vi "Ventil Setzen.vi"(8 "Error In":errorcluster caption="Fehler (Eingang)", 10 "Thermostat in %":dbl, 11 "Verbindungs-ID in":refnum<k16>) -> (0 "Error Out":errorcluster caption="Fehler (Ausgang)", 3 "Verbindungs-ID out":refnum<k16>)   [LabVIEW 2024, in "Thermostat Treiber.lvlib"]
doc: "Dieses VI sendet einen neuen Sollwert zu dem Thermotat. Der Therostat erlaubt nur Werte zweischen 0 und 100%. Wenn der Wert außerhalb des Bereiches liegt, liefert die Funktion einen fehler als Rückgabe."
uses:
  Thermostat Treiber.lvlib
  SubVIs/Simulation Share.vi
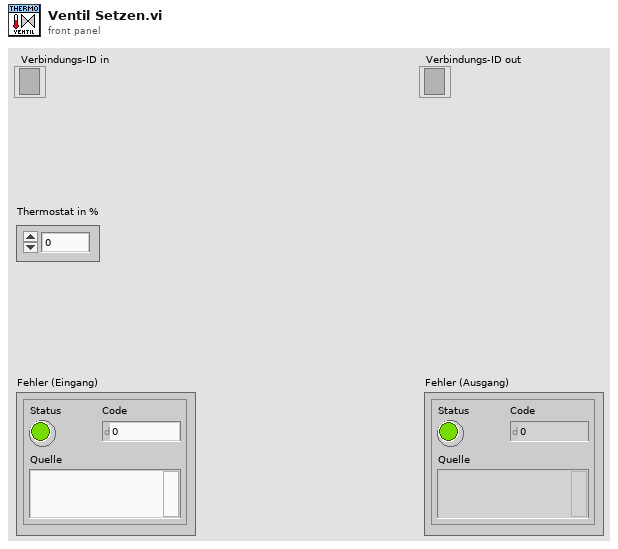
[diagram p1: front panel]
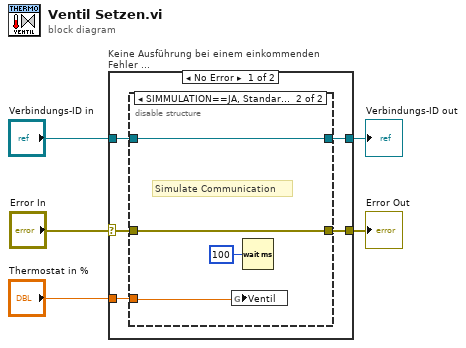
[diagram p0: block diagram]
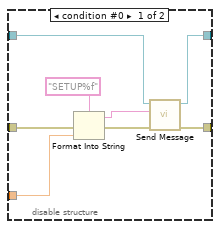
[diagram p2: hidden frame]
diagram:
  n1 = case "Keine Ausführung bei einem einkommenden Fehler ..." shown="No Error" "Error In" {
    selector: "Error In" -> [w10 w24]
    tunnel: [w7 w24] -> w4
    tunnel: "Verbindungs-ID in" -> [w9 w23]
    tunnel: [w8 w23] -> w2
    tunnel: "Thermostat in %" -> [w6 _]
    frame No Error {
      n2 = disable-structure shown="SIMMULATION==JA, Standard" {
        disable-tunnel: w10 -> [w18 w21]
        disable-tunnel: w9 -> [w17 w22]
        disable-tunnel: [w16 w22] -> w8
        disable-tunnel: [w15 w21] -> w7
        disable-tunnel: w6 -> [w12 w20]
        frame condition #0 {
          n3 = Format Into String(format string="SETUP%f" ("Nachricht"), error in=w18, w12) -> (resulting string=w13:string, error out=w14:errorcluster)  [unwired: 1 in]
          n4 = call "Send Message.vi"("Error In"=w14, "Nachricht"=w13, "Verbindungs-ID in"=w17) -> ("Error Out"=w15:errorcluster, "Verbindungs-ID out"=w16:refnum<k16>)  [unwired: 7 in]
        }
        frame condition #1 (active) {
          # "Simulate Communication"
          n5 = global write "Simulation Share.vi" "Ventil"(w20) -> ()
          n6 = Wait (ms)(milliseconds to wait=u32 100 ("Zu wartende ms")) -> ()  [unwired: 1 out]
        }
      }
    }
    frame Error {
    }
  }
  "Error Out" <- w4
  "Verbindungs-ID out" <- w2
